vi "Get_UDcluster.vi"(0 "Cluster":T3, 11 "error in (no error)":errorcluster) -> (4 "User-data cluster out":T1, 15 "error out":errorcluster)   [LabVIEW 2012]
uses:
  typedef/User Accounts.ctl
  typedef/User_Data_Cluster.ctl
panel:
  in  "User-data cluster":T1
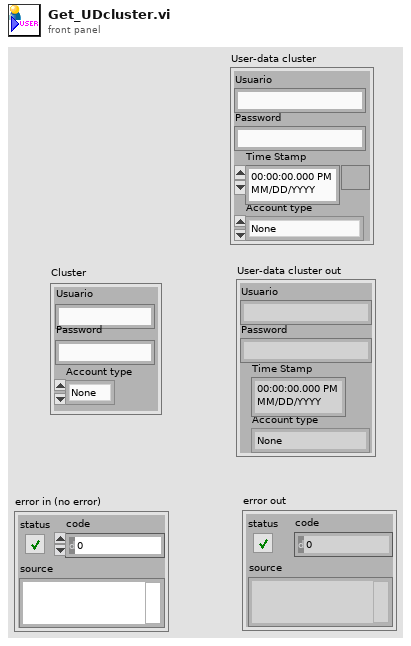
[diagram p1: front panel]
types:
  T1 = typedef "User_Data_Cluster.ctl" = cluster{"Usuario":string, "Password":string, "Account type":T2, "Time Stamp":timestamp}
  T2 = typedef "User Accounts.ctl" = enum16{"None", "User", "Admin"}
  T3 = cluster{"Usuario":string, "Password":string, "Account type":T2}
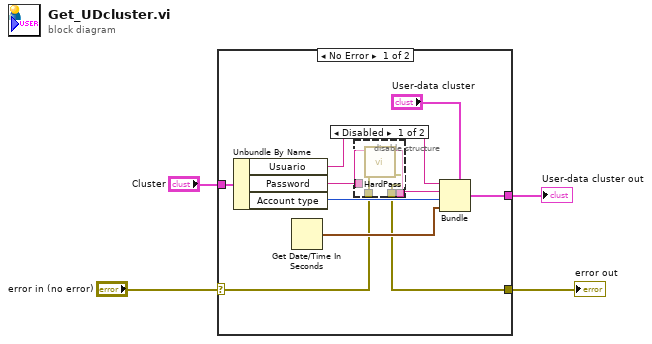
[diagram p0: block diagram]
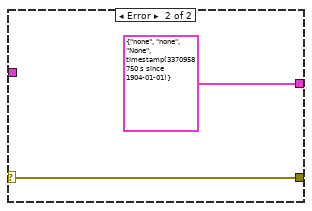
[diagram p3: hidden frame]
diagram:
  n1 = case shown="No Error" "error in (no error)" {
    selector: "error in (no error)" -> [w6 w21]
    tunnel: "Cluster" -> [w13 _]
    tunnel: [w7 T1 {"Usuario"="none", "Password"="none", "Account type"=enum."None", "Time Stamp"=timestamp(3370958750.5313764 s since 1904-01-01)} ("User-data cluster 2")] -> w3
    tunnel: [w5 w21] -> w1
    frame No Error {
      n2 = Unbundle By Name(w13) -> ("Usuario"=w12:string, "Password"=w9:string, "Account type"=w11:T2)
      n3 = Get Date/Time In Seconds() -> (seconds since 1Jan1904=w10:timestamp)
      n4 = disable-structure shown="Disabled" {
        disable-tunnel: [w18 w19] -> w14
        disable-tunnel: w9 -> [w17 w19]
        disable-tunnel: w6 -> [w16 _]
        disable-tunnel: [w15 _] -> w5
        frame Disabled {
          n5 = call "HardPass.vi"("error in (no error)"=w16, "Password"=w17) -> ("error out"=w15:errorcluster, "Password out"=w18:string)  [unwired: 8 in]
        }
        frame Enabled {
        }
      }
      n6 = Bundle(cluster="User-data cluster", "Usuario"=w12, "Password"=w14, "Account type"=w11, "Time Stamp"=w10) -> (w7:T1)
    }
    frame Error {
    }
  }
  "User-data cluster out" <- w3
  "error out" <- w1
